vi "sendHeader.vi"(8 "error in (no error)":errorcluster, 10 "MessageHeader":T1, 11 "M1M3SAL in":refnum<class "M1M3SAL.lvclass">) -> (0 "error out":errorcluster, 3 "M1M3SAL out":refnum<class "M1M3SAL.lvclass">)   [LabVIEW 2016, in "M1M3SAL.lvlib" / "M1M3SAL.lvclass"]
uses:
  M1M3SAL.lvclass
  MessageHeader.ctl
  MessageTypes.ctl
  MessageTopics.ctl
  M1M3SAL.lvlib
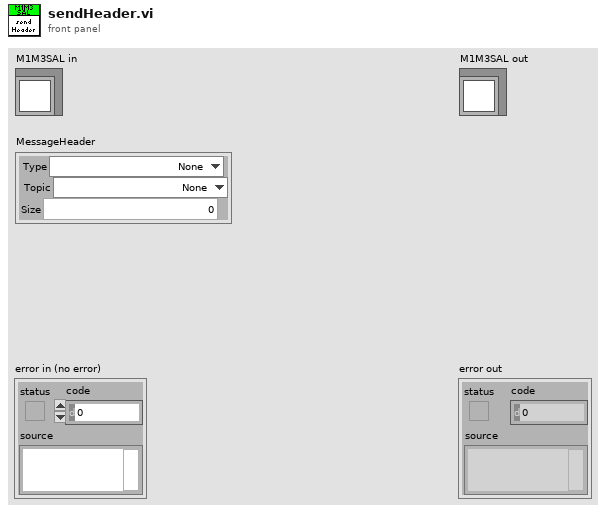
[diagram p1: front panel]
types:
  T1 = typedef "M1M3SAL.lvlib/MessageHeader.ctl" = cluster{"Type":T2, "Topic":T3, "Size":dbl}
  T2 = typedef "M1M3SAL.lvlib/MessageTypes.ctl" = enum8{"None", "PutSample", "LogEvent", "GetEvent", "IssueCommand", "CommandId", "WaitForCompletion", "AcceptCommand", "AckCommand"}
  T3 = typedef "M1M3SAL.lvlib/MessageTopics.ctl" = enum8{"None", "EnterControl", "Start", "Enable", "Disable", "Standby", "ExitControl", "AppliedSettingsMatchStart", "ErrorCode", "SettingVersions", "SummaryState"}
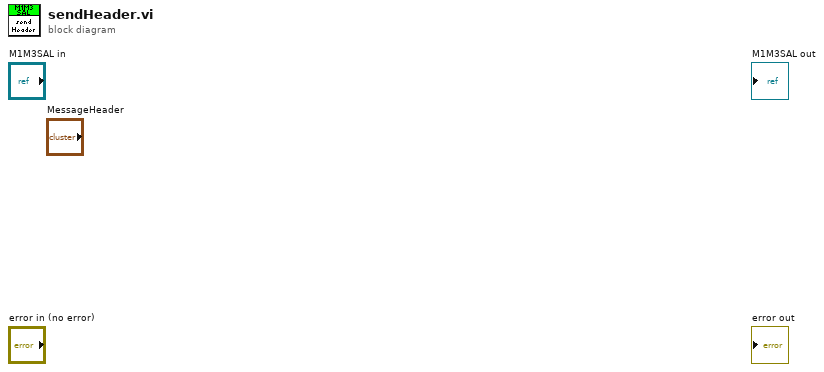
[diagram p0: block diagram]
diagram:
